vi "EMG.vi"() -> ()   [LabVIEW 2017]
uses:
  <vilib>/addons/Biomedical/NI_BMTK_Measurements.lvlib
  <vilib>/addons/Biomedical/Biosignal Measurements/EMG/EMG Mean Power Frequency (Waveform).vi
  <vilib>/addons/Biomedical/Biosignal Measurements/EMG/EMG Median Power Frequency (Waveform).vi
  <vilib>/addons/Biomedical/Biosignal Measurements/Biosignal Preprocessing/subVIs/bmt_Window Info_Waveform.ctl
panel:
  out "MDF":cluster{"t0":dbl, "dt":dbl, "frequency":dbl[]}
  out "MNF":cluster{"t0":dbl, "dt":dbl, "frequency":dbl[]}
  out "RMS value":waveform(dbl)
  in  "EMG":waveform(dbl)
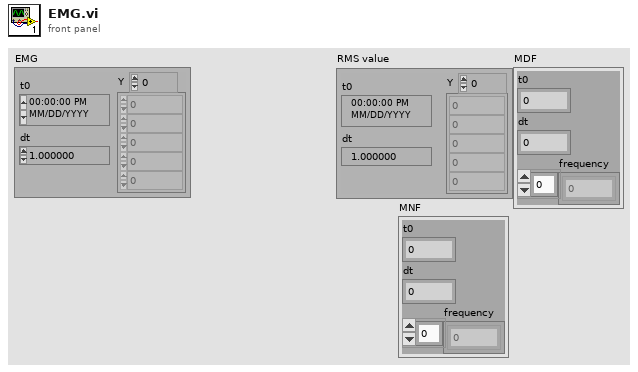
[diagram p1: front panel]
types:
  T1 = typedef "NI_BMTK_Measurements.lvlib/bmt_Window Info_Waveform.ctl" = cluster{"time":dbl}
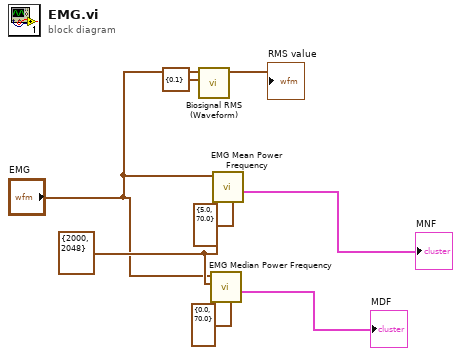
[diagram p0: block diagram]
diagram:
  w6 = cluster{"time steps":i32, "frequency bins":i32} {"time steps"=2000, "frequency bins"=2048} ("time-freq sampling info")
  n1 = call <vilib>:"Biosignal RMS (Waveform).vi"("window info"=T1 {"time"=0.1}, "biosignal"="EMG") -> ("RMS value"=→"RMS value":waveform(dbl))  [unwired: 8 in, 1 out]
  n2 = call-poly <vilib>:"EMG Median Power Frequency.vi"("trimmed percentage"=cluster{"upper":dbl, "lower":dbl} {"upper"=0.0, "lower"=70.0}, "time-freq sampling info"=w6, "EMG"="EMG") -> ("MDF"=→"MDF":cluster{"t0":dbl, "dt":dbl, "frequency":dbl[]})  [unwired: 5 in, 3 out]
  n3 = call-poly <vilib>:"EMG Mean Power Frequency.vi"("trimmed percentage"=cluster{"upper":dbl, "lower":dbl} {"upper"=5.0, "lower"=70.0}, "time-freq sampling info"=w6, "EMG"="EMG") -> ("MNF"=→"MNF":cluster{"t0":dbl, "dt":dbl, "frequency":dbl[]})  [unwired: 5 in, 3 out]
